vi "Bivariate_Gaussian_Matrix.vi"(8 "correlation":dbl, 9 "B":cluster{"mean":dbl, "sd":dbl}, 10 "A":cluster{"mean":dbl, "sd":dbl}, 11 "Data":cluster{"Xa":dbl, "Xa B":dbl}) -> (0 "Sigma Array":T1, 1 "Mahalanobis Distance":dbl, 2 "Data":T1, 3 "P":dbl)   [LabVIEW 2017]
uses:
  <vilib>/Analysis/Matrix/Datatypes/RealMatrix.ctl
  <vilib>/Analysis/baseanly.llb/Real Determinant.vi
  <vilib>/Analysis/baseanly.llb/Real Inverse Matrix.vi
  <vilib>/Analysis/Matrix/Numeric/Multiply/Multiply - RM,RM.vi
  <vilib>/Analysis/Matrix/Numeric/Multiply/Multiply - R,RM.vi
  <vilib>/Analysis/Matrix/Numeric/Exponential/Exponential - RM.vi
  <vilib>/Analysis/Matrix/Numeric/Multiply/Multiply - RM,R.vi
  <vilib>/Analysis/NI_AALBase.lvlib
  <vilib>/Analysis/Matrix/NI_Matrix.lvlib
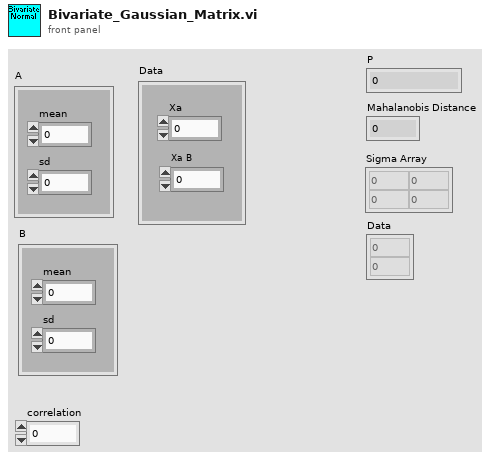
[diagram p1: front panel]
types:
  T1 = typedef "NI_Matrix.lvlib/RealMatrix.ctl" = dbl[][]
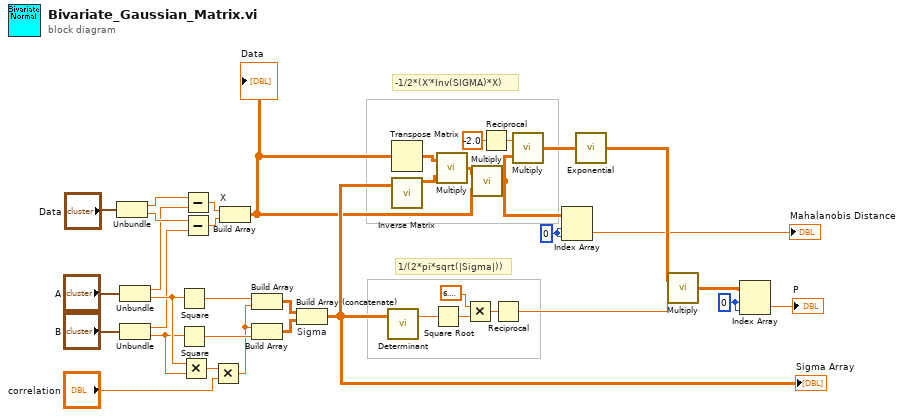
[diagram p0: block diagram]
diagram:
  w3 = 0 ("index (row)")
  w5 = 0 ("index (row)")
  # "-1/2*(X'*Inv(SIGMA)*X)"
  # "1/(2*pi*sqrt(|Sigma|))"
  n1 = Unbundle("Data") -> ("Xa"=w24:dbl, "Xa B"=w23:dbl)
  n2 = Unbundle("A") -> ("mean"=w22:dbl, "sd"=w32:dbl)
  n3 = Unbundle("B") -> ("mean"=w21:dbl, "sd"=w31:dbl)
  n4 = Square(x=w32) -> (x^2=w38:dbl)
  n5 = Square(x=w31) -> (x^2=w37:dbl)
  n6 = Multiply(x=w32, y=w31) -> (x*y=w30:dbl)
  n7 = Subtract(x=w24, y=w22) -> (x-y=w26:dbl)
  n8 = Subtract(x=w23, y=w21) -> (x-y=w25:dbl)
  n9 = Multiply(x=w30, y="correlation") -> (x*y=w28:dbl)
  n10 = Build Array "X"(w26, w25) -> (w10:T1)
  "Data" <- w10
  n11 = Build Array(w38, w28) -> (w36:T1)
  n12 = Build Array(w28, w37) -> (w35:T1)
  n13 = Build Array (concatenate) "Sigma"(w36, w35) -> (w14:T1)
  "Sigma Array" <- w14
  n14 = call-poly <vilib>:"Determinant.vi"("Input Matrix"=w14) -> ("determinant"=w20:dbl)  [unwired: 1 in, 1 out]
  n15 = Transpose Matrix(1:w10) -> (0:w13:T1)
  n16 = call-poly <vilib>:"Inverse Matrix.vi"("Input Matrix"=w14) -> ("Inverse Matrix"=w12:T1)  [unwired: 1 in, 1 out]
  n17 = Square Root(x=w20) -> (sqrt(x)=w19:dbl)
  n18 = call-poly <vilib>:"Multiply.vi"("Real Matrix B"=w12, "Real Matrix A"=w13) -> ("A * B"=w11:T1)
  n19 = Multiply(x=6.283185307179586, y=w19) -> (x*y=w17:dbl)
  n20 = call-poly <vilib>:"Multiply.vi"("Real Matrix B"=w10, "Real Matrix A"=w11) -> ("A * B"=w2:T1)
  n21 = Reciprocal(x=-2.0) -> (1/x=w15:dbl)
  n22 = Reciprocal(x=w17) -> (1/x=w7:dbl)
  n23 = call-poly <vilib>:"Multiply.vi"("Real Matrix A"=w2, "Real Scalar c"=w15) -> ("c * A"=w9:T1)
  n24 = Index Array(array=w2, index (row)=w3, index (col)=w3) -> (element=→"Mahalanobis Distance":dbl)
  n25 = call-poly <vilib>:"Exponential.vi"("Real Matrix A"=w9) -> ("e^A"=w8:T1)
  n26 = call-poly <vilib>:"Multiply.vi"("Real Scalar c"=w7, "Real Matrix A"=w8) -> ("A * c"=w6:T1)
  n27 = Index Array(array=w6, index (row)=w5, index (col)=w5) -> (element=→"P":dbl)
